vi "Log Folder.vi"(8 "error in (no error)":errorcluster, 11 "Event Reporter Module in":refnum<class "Event Reporter Module.lvclass">) -> (0 "error out":errorcluster, 2 "Log Folder":path, 3 "Event Reporter Module out":refnum<class "Event Reporter Module.lvclass">)   [LabVIEW 2020, in "Volatus.lvlib" / "Event Reporter Module.lvclass"]
uses:
  Event Reporter Module.lvclass
  Event Reporter Module.lvclass/Event Reporter Module.ctl
  Module/Module.lvclass
  lv-cdm/CDM-Config/Config Element/Config Element.lvclass
  C:/dev/lv20CE/relink/lv-volatus/Volatus/Module/Module.lvclass
  C:/dev/lv20CE/relink/lv-volatus/Volatus/Event Reporter Module/Event Reporter Module.lvclass
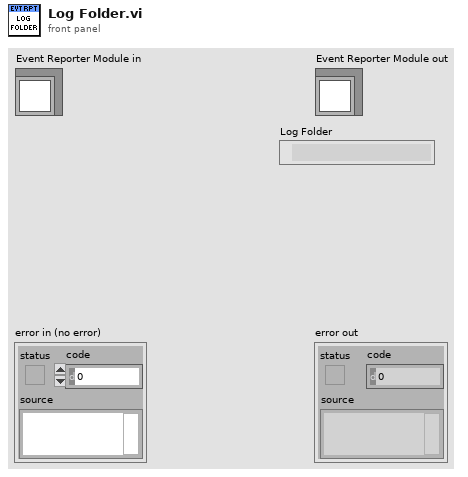
[diagram p1: front panel]
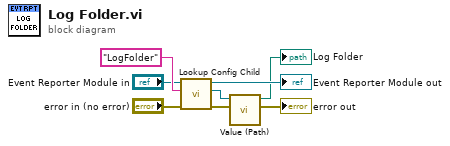
[diagram p0: block diagram]
diagram:
  n1 = call "Lookup Config Child.vi"("error in (no error)"="error in (no error)", "Name"="LogFolder", "Module in"="Event Reporter Module in") -> ("error out"=w4:errorcluster, "Config Child"=w7:refnum<class "Config Element.lvclass">, "Module out"=→"Event Reporter Module out":refnum<class "Event Reporter Module.lvclass">)  [unwired: 5 in, 1 out]
  n2 = call "Value (Path).vi"("error in (no error)"=w4, "Config Element in"=w7) -> ("error out"=→"error out":errorcluster, "Path Value"=→"Log Folder":path)  [unwired: 8 in]
